vi "Multiple Connections - Server - UDP.vi"() -> ()   [LabVIEW 2011]
doc: "Demonstrates how to establish multiple connections and place them in a queue to be serviced. As connections are made, it sends the current date and time via TCP to all Client VIs that connect to it.\n\nThis VI has two parts -- a loop that listens for each client to connect, and a loop that sends the date and time to each connection in the queue.\n\n<B>Note:</B> Use this VI with Multiple Connections - Client 1.vi and Multiple Connections - Client 2.vi."
panel:
  in  "Remote Port":u16=61557
  in  "Local Port":u16=61556
  in  "stop":bool
  out "# of Connections":i32
  in  "empty":refnum<k5>[](array[refnum])
  in  "empty":refnum<k5>[](array[refnum])
  in  "Port":u16=6341
  # "Instructions:\n1. Open the Multiple Connections - Client 1 and Client 2 VIs.\n2. Run this VI first.\n3. Run the Client VIs second and follow the instructions on their front panels.\n4. Stop This VI.  The Client VIs will stop on their own when they time out."
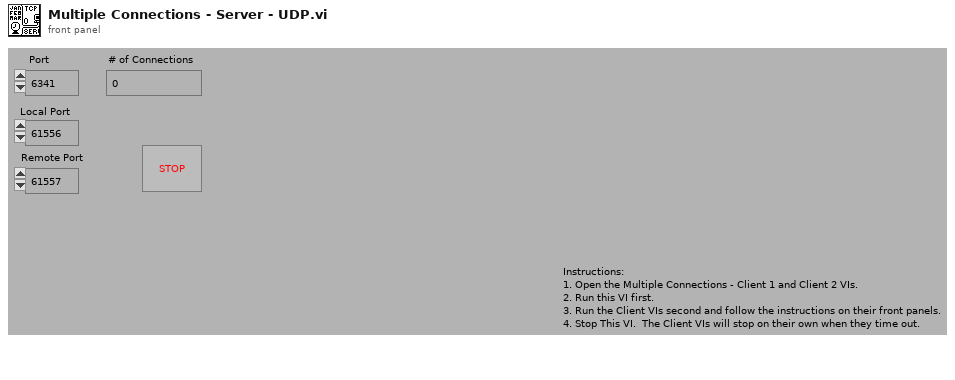
[diagram p1: front panel]
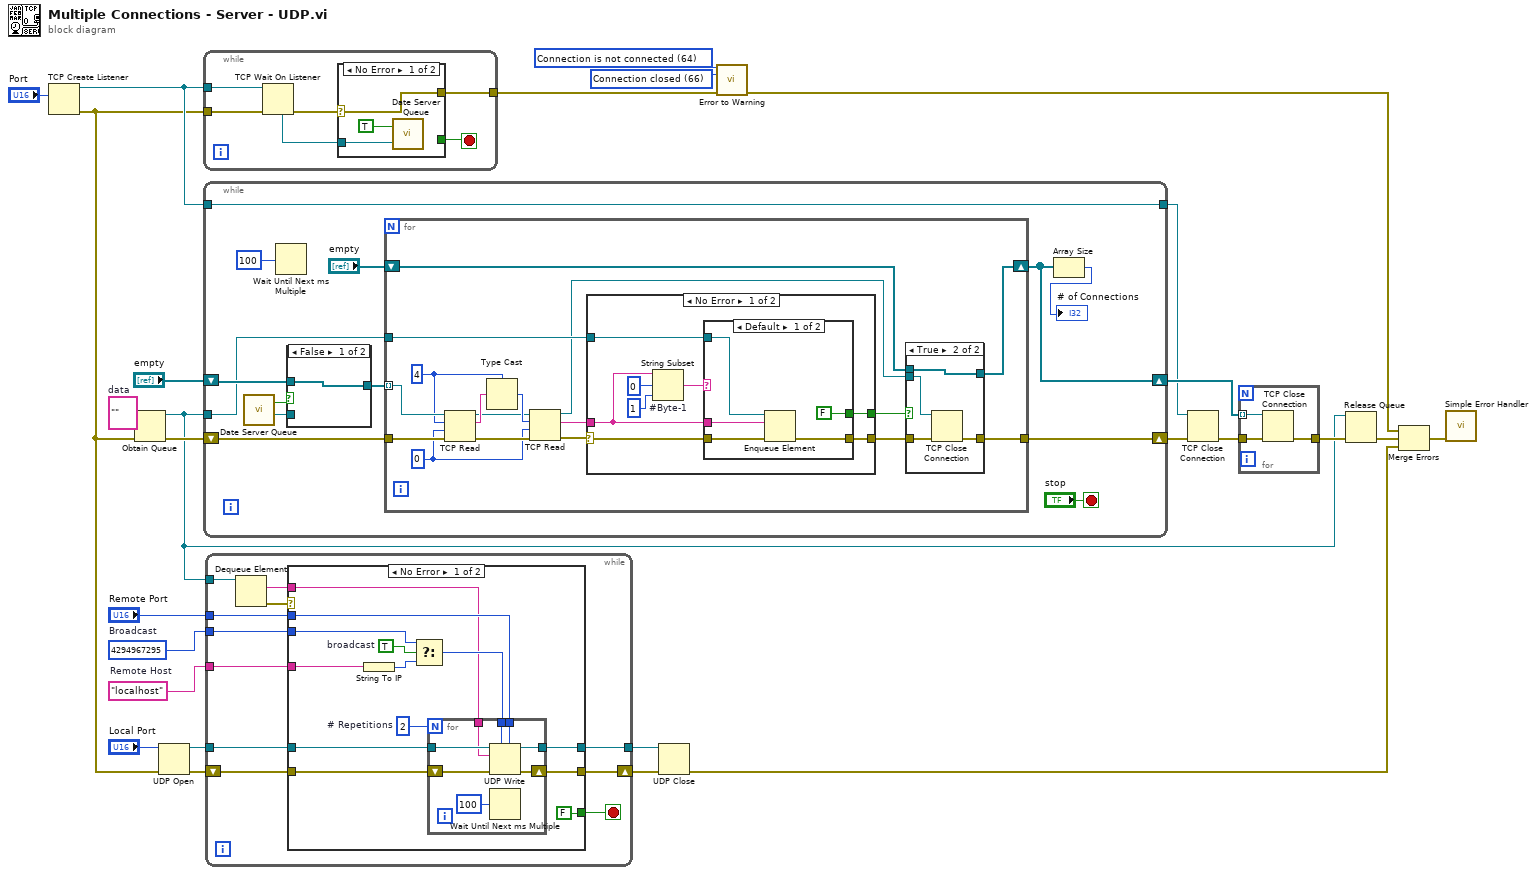
[diagram p0: block diagram]
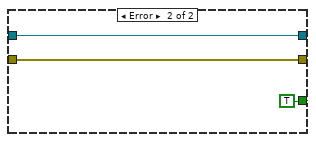
[diagram p2: hidden frame]
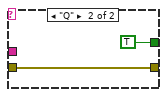
[diagram p3: hidden frame]
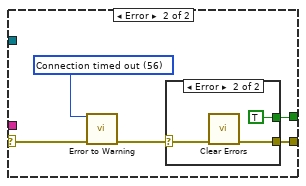
[diagram p4: hidden frame]
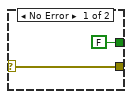
[diagram p5: hidden frame]
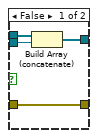
[diagram p6: hidden frame]
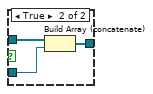
[diagram p7: hidden frame]
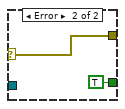
[diagram p8: hidden frame]
diagram:
  w6 = "localhost"  # Remote Host
  w5 = u32 4294967295  # Broadcast
  w15 = ""  # data
  w21 = 66 items=["No Error", "Argument Error", "Memory Full", "Out of Zone", "End of File", "File Already Open", "Generic File IO Error", "File Not Found", "File Permission Error", "Disk Full", "Duplicate Path", "Too Many Files Open", "Not Enabled", "Resource File Not Found", "Cannot Add Resource", "Resource Not Found", "Image Not Found", "Image Memory Error", "Pen Does Not Exist", "Config Bad Type", "Config Token Not Found", "Config Parse Error", "Config Memory Error", "Bad External Code Format", "Bad External Code Offset", "External Code Not Present", "Null Window", "Destroy Window Mixup", "Null Menu", "Print Aborted", "Bad Print Record", "Print Driver Error", "Windows Error During Print", "Memory Error During Print", "Print Dialog Error", "Generic Print Error", "Invalid Device Refnum", "Device Not Found", "Device Parameter Error", "Device Unit Error", "Can't Open Device", "Device Call Aborted", "Generic Error", "Cancelled By User", "Object ID Too Low", "Object ID Too High", "Object Not In Heap", "Unknown Heap", "Bad DefProc ID", "DefProc Not In Table", "Message Out Of Range", "Null Method", "Unknown Message", "Manager Call Not Supported", "Bad address", "Connection In progress", "Connection timed out", "Connection is already in progress", "Network attribute not supported", "Network error", "Address in use", "System out of memory", "Connection aborted", "Connection refused", "Connection is not connected", "Connection is already connected", "Connection closed", "Initialize error (interapplication manager)", "Bad occurrence", "Wait on unbound occurrence handler", "Occurrence queue overflow", "Bad path", "Semaphore not signaled", "Unrecognized type (interapplication manager)"] ("2nd Error to Convert")
  w22 = 64 items=["No Error", "Argument Error", "Memory Full", "Out of Zone", "End of File", "File Already Open", "Generic File IO Error", "File Not Found", "File Permission Error", "Disk Full", "Duplicate Path", "Too Many Files Open", "Not Enabled", "Resource File Not Found", "Cannot Add Resource", "Resource Not Found", "Image Not Found", "Image Memory Error", "Pen Does Not Exist", "Config Bad Type", "Config Token Not Found", "Config Parse Error", "Config Memory Error", "Bad External Code Format", "Bad External Code Offset", "External Code Not Present", "Null Window", "Destroy Window Mixup", "Null Menu", "Print Aborted", "Bad Print Record", "Print Driver Error", "Windows Error During Print", "Memory Error During Print", "Print Dialog Error", "Generic Print Error", "Invalid Device Refnum", "Device Not Found", "Device Parameter Error", "Device Unit Error", "Can't Open Device", "Device Call Aborted", "Generic Error", "Cancelled By User", "Object ID Too Low", "Object ID Too High", "Object Not In Heap", "Unknown Heap", "Bad DefProc ID", "DefProc Not In Table", "Message Out Of Range", "Null Method", "Unknown Message", "Manager Call Not Supported", "Bad address", "Connection In progress", "Connection timed out", "Connection is already in progress", "Network attribute not supported", "Network error", "Address in use", "System out of memory", "Connection aborted", "Connection refused", "Connection is not connected", "Connection is already connected", "Connection closed", "Initialize error (interapplication manager)", "Bad occurrence", "Wait on unbound occurrence handler", "Occurrence queue overflow", "Bad path", "Semaphore not signaled", "Unrecognized type (interapplication manager)"] ("1st Error to Convert")
  n1 = TCP Create Listener(10:"Port") -> (0:w3:errorcluster, 3:w24:refnum<k5>)  [unwired: 1 in, 4 out]
  n2 = Obtain Queue(element data type=w15, error in (no error)=w3) -> (queue out=w11:refnum<queue>, error out=w16:errorcluster)  [unwired: 3 in, 1 out]
  n3 = UDP Open(8:w3, 11:"Local Port") -> (port=w10:refnum<k16>, 0:w9:errorcluster)  [unwired: 4 out]
  n4 = while "Listen loop.  Append new connections to a synchronized queue." {
    tunnel: w24 -> [w32]
    tunnel: w3 -> [w33]
    tunnel: [w28] -> w23
    stop <- w29 stop-if-true
    n5 = TCP Wait On Listener(8:w33, 11:w32) -> (0:w30:errorcluster, 4:w31:refnum<k5>)  [unwired: 5 out]
    n6 = case shown="No Error" w30 {
      selector: w30 -> [w34 w37]
      tunnel: w31 -> [w35 _]
      tunnel: [_ TRUE] -> w29
      tunnel: [w34 w37] -> w28
      frame No Error {
        n7 = call "Date Server Queue.vi"("new value"=w35, "set queue? (F: de-queue)"=TRUE) -> ()  [unwired: 2 out]
      }
      frame Error {
      }
    }
  }
  n8 = while {
    shift-left: "empty" -> [w49]
    shift-right: [w46] -> w27
    tunnel: w24 -> [w44]
    tunnel: [w44] -> w25
    shift-right: [w41] -> w14
    shift-left: w16 -> [w42]
    tunnel: w11 -> [w40]
    stop <- "stop" stop-if-true
    n9 = call "Date Server Queue.vi"() -> ("value"=w51:refnum<k5>, "valid?"=w50:bool)  [unwired: 2 in]
    n10 = Wait Until Next ms Multiple(millisecond multiple=u32 100) -> ()  [unwired: 1 out]
    n11 = case shown="False" w50 {
      tunnel: w51 -> [_ w105]
      tunnel: w49 -> [w102 w104]
      tunnel: [w102 w103] -> w48
      frame False {
      }
      frame True {
        n12 = Build Array (concatenate)(w104, w105) -> (w103:refnum<k5>[])
      }
    }
    n13 = for {
      tunnel: w48 -> [w65] mode=indexing
      shift-right: [w67] -> w46
      shift-left: "empty" -> [w68]
      tunnel: [w66] -> w41
      tunnel: w42 -> [w64]
      tunnel: w40 -> [w63]
      w56 = 0 ("timeout ms (25000)")
      w58 = 4
      n14 = TCP Read(connection ID=w65, bytes to read=w58, error in (no error)=w64, 9:w56) -> (connection ID out=w54:refnum<k5>, data out=w57:string, error out=w60:errorcluster)  [unwired: 1 out]
      n15 = Type Cast(type=w58, x=w57) -> (*(type *) &x=w55:i32)
      n16 = TCP Read(connection ID=w54, bytes to read=w55, error in (no error)=w60, 9:w56) -> (connection ID out=w52:refnum<k5>, data out=w53:string, error out=w59:errorcluster)  [unwired: 1 out]
      n17 = case shown="No Error" w59 {
        selector: w59 -> [w69 w87]
        tunnel: [w72 w85] -> w62
        tunnel: w63 -> [w73 _]
        tunnel: [w71 w84] -> w61
        tunnel: w53 -> [w70 _]
        frame No Error {
          n18 = String Subset "#Byte-1"(string=w70, offset (0)=0, length (rest)=1 ("length (rest)")) -> (substring=w74:string)
          n19 = case shown="Default" w74 {
            tunnel: w70 -> [w81 _]
            tunnel: w69 -> [w80 w83]
            tunnel: [w78 w83] -> w72
            tunnel: w73 -> [w79 _]
            tunnel: [FALSE TRUE] -> w71
            frame Default {
              n20 = Enqueue Element(queue=w79, element=w81, error in (no error)=w80) -> (error out=w78:errorcluster)  [unwired: 1 in, 2 out]
            }
            frame "Q" {
            }
          }
        }
        frame Error {
          w88 = 56 items=["No Error", "Argument Error", "Memory Full", "Out of Zone", "End of File", "File Already Open", "Generic File IO Error", "File Not Found", "File Permission Error", "Disk Full", "Duplicate Path", "Too Many Files Open", "Not Enabled", "Resource File Not Found", "Cannot Add Resource", "Resource Not Found", "Image Not Found", "Image Memory Error", "Pen Does Not Exist", "Config Bad Type", "Config Token Not Found", "Config Parse Error", "Config Memory Error", "Bad External Code Format", "Bad External Code Offset", "External Code Not Present", "Null Window", "Destroy Window Mixup", "Null Menu", "Print Aborted", "Bad Print Record", "Print Driver Error", "Windows Error During Print", "Memory Error During Print", "Print Dialog Error", "Generic Print Error", "Invalid Device Refnum", "Device Not Found", "Device Parameter Error", "Device Unit Error", "Can't Open Device", "Device Call Aborted", "Generic Error", "Cancelled By User", "Object ID Too Low", "Object ID Too High", "Object Not In Heap", "Unknown Heap", "Bad DefProc ID", "DefProc Not In Table", "Message Out Of Range", "Null Method", "Unknown Message", "Manager Call Not Supported", "Bad address", "Connection In progress", "Connection timed out", "Connection is already in progress", "Network attribute not supported", "Network error", "Address in use", "System out of memory", "Connection aborted", "Connection refused", "Connection is not connected", "Connection is already connected", "Connection closed", "Initialize error (interapplication manager)", "Bad occurrence", "Wait on unbound occurrence handler", "Occurrence queue overflow", "Bad path", "Semaphore not signaled", "Unrecognized type (interapplication manager)"] ("1st Error to Convert")
          n21 = call <vilib>:"Error to Warning.vi"("1st Error to Convert"=w88, "error in"=w87) -> ("warning out"=w86:errorcluster)  [unwired: 13 in]
          n22 = case shown="Error" w86 {
            selector: w86 -> [w90 w93]
            tunnel: [w90 w92] -> w85
            tunnel: [FALSE TRUE] -> w84
            frame No Error {
            }
            frame Error {
              n23 = call <vilib>:"Clear Errors.vi"("error in (no error)"=w93) -> ("error out"=w92:errorcluster)  [unwired: 6 in]
            }
          }
        }
      }
      n24 = case shown="True" w61 {
        tunnel: w68 -> [w97 w101]
        tunnel: [w96 w101] -> w67
        tunnel: w62 -> [w95 w100]
        tunnel: [w95 w99] -> w66
        tunnel: w52 -> [w94 w98]
        frame False {
          n25 = Build Array (concatenate)(w97, w94) -> (w96:refnum<k5>[])
        }
        frame True {
          n26 = TCP Close Connection(connection ID=w98, error in (no error)=w100) -> (error out=w99:errorcluster)  [unwired: 2 out]
        }
      }
    }
    n27 = Array Size(array=w46) -> (size(s)=→"# of Connections":i32)
  }
  n28 = while {
    tunnel: w11 -> [w116]
    tunnel: w10 -> [w113]
    tunnel: "Remote Port" -> [w111]
    tunnel: w6 -> [w110]
    tunnel: w5 -> [w109]
    tunnel: [w108] -> w4
    shift-right: [w107] -> w2
    shift-left: w9 -> [w112]
    stop <- w106 stop-if-true
    n29 = Dequeue Element(queue=w116) -> (element=w114:string, error out=w115:errorcluster)  [unwired: 2 in, 2 out]
    n30 = case shown="No Error" w115 {
      tunnel: w114 -> [w120 _]
      tunnel: w113 -> [w125 w140]
      tunnel: w112 -> [w124 w139]
      tunnel: [w119 w139] -> w107
      tunnel: w111 -> [w123 _]
      tunnel: w110 -> [w122 _]
      tunnel: w109 -> [w121 _]
      tunnel: [w118 w140] -> w108
      tunnel: [FALSE TRUE] -> w106
      frame No Error {
        w126 = 2  # # Repetitions
        w129 = TRUE  # broadcast
        n31 = String To IP(1:w122) -> (0:w128:u32)
        n32 = Select(t=w121, s=w129, f=w128) -> (s? t:f=w127:u32)
        n33 = for {
          N: w126 -> [_]
          tunnel: w125 -> [w135]
          tunnel: w127 -> [w137]
          tunnel: w123 -> [w136]
          shift-right: [w133] -> w119
          shift-left: w124 -> [w134]
          tunnel: [w132] -> w118
          tunnel: w120 -> [w130]
          n34 = UDP Write(address=w137, port or service name=w136, connection ID=w135, data in=w130, 8:w134) -> (error out=w133:errorcluster, 3:w132:refnum<k16>)  [unwired: 1 out]
          n35 = Wait Until Next ms Multiple(millisecond multiple=u32 100) -> ()  [unwired: 1 out]
        }
      }
      frame Error {
      }
    }
  }
  n36 = UDP Close(connection ID=w4, 8:w2) -> (error out=w8:errorcluster)  [unwired: 1 out]
  n37 = call <vilib>:"Error to Warning.vi"("1st Error to Convert"=w22, "2nd Error to Convert"=w21, "error in"=w23) -> ("warning out"=w17:errorcluster)  [unwired: 2 in, 10 out]
  n38 = TCP Close Connection(connection ID=w25, error in (no error)=w14) -> (error out=w18:errorcluster)  [unwired: 2 out]
  n39 = for {
    tunnel: w27 -> [w143] mode=indexing
    tunnel: [w142] -> w13
    tunnel: w18 -> [w141]
    n40 = TCP Close Connection(connection ID=w143, error in (no error)=w141) -> (error out=w142:errorcluster)  [unwired: 2 out]
  }
  n41 = Release Queue(queue=w11, error in (no error)=w13) -> (error out=w12:errorcluster)  [unwired: 1 in, 2 out]
  n42 = Merge Errors(w17, w12, w8) -> (w20:errorcluster)
  n43 = call <vilib>:"Simple Error Handler.vi"("error in (no error)"=w20) -> ()  [unwired: 1 in, 8 out]
